vi "initialize.vi"(0 "MoAgSy_GPG":refnum<class "MoAgSy_GPG.lvclass">, 3 "initializationData":variant, 5 "error in (no error)":errorcluster, 7 "binaryString":string, 8 "I8 Array":i8[](array[numeric]), 9 "prependSize? (T)":bool, 11 "byteOrder (0:big-endian, network order)":T1(ring)) -> (14 "dup MoAgSy_GPG":refnum<class "MoAgSy_GPG.lvclass">, 17 "found":bool, 19 "error out":errorcluster)   [LabVIEW 2009, in "MoAgSy.lvlib" / "MoAgSy_GPG.lvclass"]
doc: "This is a dynamic dispatch VI to be implemented by child classes to initialize their attributes.\n\n<B>Recommendation:</B> Use Variant for initialization data."
uses:
  MoAgSy_GPG.lvclass
  HGF_GPG/HGF_GPG.lvclass/HGF_GPG.lvclass
  MoAgSy_GPG.lvclass/MoAgSy_GPG.ctl
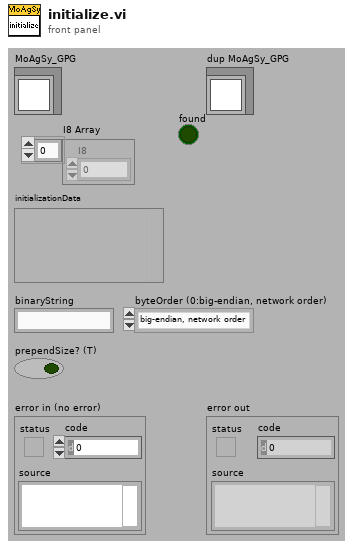
[diagram p1: front panel]
types:
  T1 = enum16{"big-endian, network order", "native, host order", "little-endian"}
  T2 = enum32{"invalid app kind", "Development System", "Run Time System", "Student Edition", "Embedded LabVIEW", "Evaluation", "Custom"}
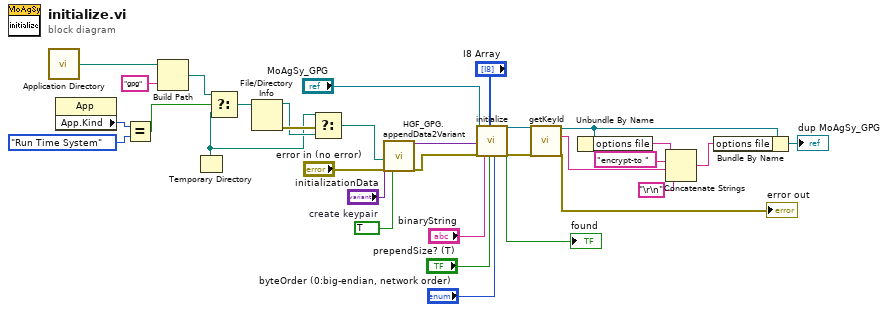
[diagram p0: block diagram]
diagram:
  w24 = TRUE  # create keypair
  n1 = call <vilib>:"Application Directory.vi"() -> ("Application Directory"=w6:path)
  n2 = property class="App"() -> ("App.Kind"=w8:T2)  [unwired: 2 in, 2 out]
  n3 = Equal?(x=w8, y=T2."Run Time System" ("Application:Kind")) -> (x = y?=w11:bool)
  n4 = Build Path(base path=w6, name or relative path="gpg") -> (appended path=w10:path)
  n5 = Temporary Directory() -> (w2:path)
  n6 = Select(t=w10, s=w11, f=w2) -> (s? t:f=w5:path)
  n7 = File/Directory Info(path=w5) -> (path out=w3:path, error out=w4:errorcluster)  [unwired: 1 in, 5 out]
  n8 = Select(t=w2, s=w4, f=w3) -> (s? t:f=w1:path)
  n9 = call "HGF_GPG.appendData2Variant.vi"("initData"="initializationData", "GPG-folder"=w1, "create keypair"=w24, "error in (no error)"="error in (no error)") -> ("dup initData"=w26:variant, "error out"=w25:errorcluster)  [unwired: 7 in, 7 out]
  n10 = call-parent "initialize.vi"("HGF_GPG"="MoAgSy_GPG", "initializationData"=w26, "error in (no error)"=w25, "binaryString"="binaryString", "I8 Array"="I8 Array", "prependSize? (T)"="prependSize? (T)", "byteOrder (0:big-endian, network order)"="byteOrder (0:big-endian, network order)") -> ("dup HGF_GPG"=w21:refnum<class "MoAgSy_GPG.lvclass">, "found"=→"found":bool, "error out"=w20:errorcluster)  [unwired: 10 out]
  n11 = call-dynamic "getKeyId.vi"("HGF_GPG.lvclass in"=w21, "error in (no error)"=w20) -> ("HGF_GPG.lvclass out"=w18:refnum<class "MoAgSy_GPG.lvclass">, "Key-ID"=w13:string, "error out"=→"error out":errorcluster)  [unwired: 15 out]
  n12 = Unbundle By Name(w18) -> ("options file"=w16:string)
  n13 = Concatenate Strings(w16, "encrypt-to " ("string"), w13, "\r\n") -> (w15:string)
  n14 = Bundle By Name(cluster=w18, "options file"=w15) -> (→"dup MoAgSy_GPG":refnum<class "MoAgSy_GPG.lvclass">)
